vi "act_iso_leds.vi"() -> (0 "iso_led_2":bool, 1 "iso_led_1":bool)   [LabVIEW 2018]
uses:
  <vilib>/rvi/DataTransferAndStorage/Container/Common/niFpgaContainerExecOnDevCompGetState.vi
  <vilib>/rvi/Emulation/niFpgaEmulationIsFPGAContextNoSignature.vi
  <vilib>/rvi/DataTransferAndStorage/Container/Common/niFpgaContainerGetUniqueNameForEmu.vi
  <vilib>/rvi/Memory/Memory_Emulation/niFpgaMemoryEmulationCacheClearOnFirstRun.vi
  <vilib>/rvi/Memory/Memory_Emulation/nirvimemoryEmulationManagerCache_MakeExclusive.vi
  <vilib>/rvi/Memory/Memory_Emulation/niFpgaMemoryEmulationValidateCache.vi
  <vilib>/rvi/Memory/Memory_Emulation/nirvimemoryEmulationManagerCache_InsertValue.vi
  <vilib>/Utility/error.llb/Clear Errors.vi
  <vilib>/rvi/Memory/Memory_Emulation/nirvimemoryEmulationManagerCache_ReleaseExclusive.vi
  <vilib>/rvi/Memory/Memory_Emulation/nirvimemoryEmulationManagerCache_GetValue.vi
  <vilib>/rvi/Memory/Memory_Emulation/nirvimemoryEmulationManagerCache_SetValue.vi
  <vilib>/rvi/Emulation/niFpgaProcessEmulError.vi
  <vilib>/rvi/Emulation/niFpgaSctlEmulationGetInTimedLoop.vi
  <vilib>/rvi/eio/common/nirviEmuTemplateMethod_errors.vi
  <vilib>/rvi/DataTransferAndStorage/Container/XNode/niFpgaContainer.xnode
  <vilib>/rvi/DataTransferAndStorage/Register/Emulation/niFpgaRegisterEmulationRefIn.vi
  <vilib>/eio/EIONode/EIONode.xnode
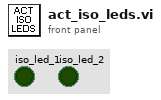
[diagram p1: front panel]
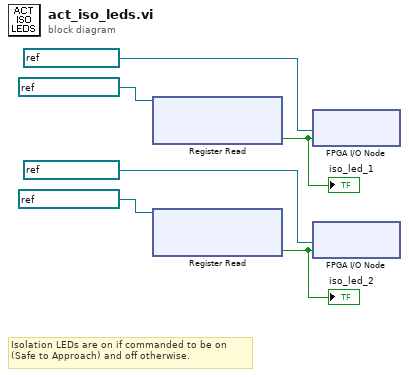
[diagram p0: block diagram]
diagram:
  # "Isolation LEDs are on if commanded to be on \n(Safe to Approach) and off otherwise."
  n1 = xnode "Register Read"("Register In"=refnum<k21> "REG_iso_led_1") -> ("Data"=w1:bool)  [unwired: 1 out]
  "iso_led_1" <- w1
  n2 = xnode "Register Read"("Register In"=refnum<k21> "REG_iso_led_2") -> ("Data"=w2:bool)  [unwired: 1 out]
  "iso_led_2" <- w2
  n3 = xnode "FPGA I/O Node"("I/O Item"=w1, "FPGA I/O In"=refnum<k21> "Mod2/DIO16") -> ()  [unwired: 1 out]
  n4 = xnode "FPGA I/O Node"("I/O Item"=w2, "FPGA I/O In"=refnum<k21> "Mod2/DIO17") -> ()  [unwired: 1 out]
